vi "senser.vi"(1 "read buffer":string) -> (0 "输出簇":T1)   [LabVIEW 2014]
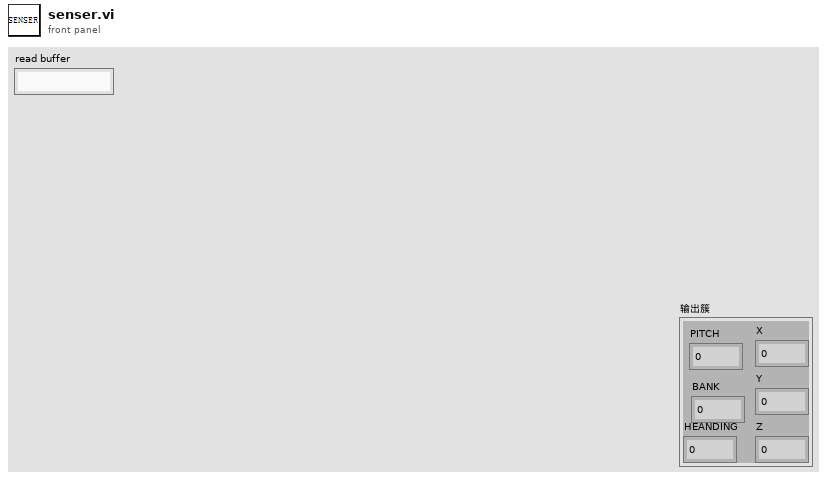
[diagram p1: front panel]
types:
  T1 = cluster{"PITCH":i32, "BANK":i32, "HEANDING":i32, "X":i32, "Y":i32, "Z":i32}
  T2 = cluster{"32位整型":i32, "32位整型":i32, "32位整型":i32, "32位整型":i32, "32位整型":i32, "32位整型":i32}
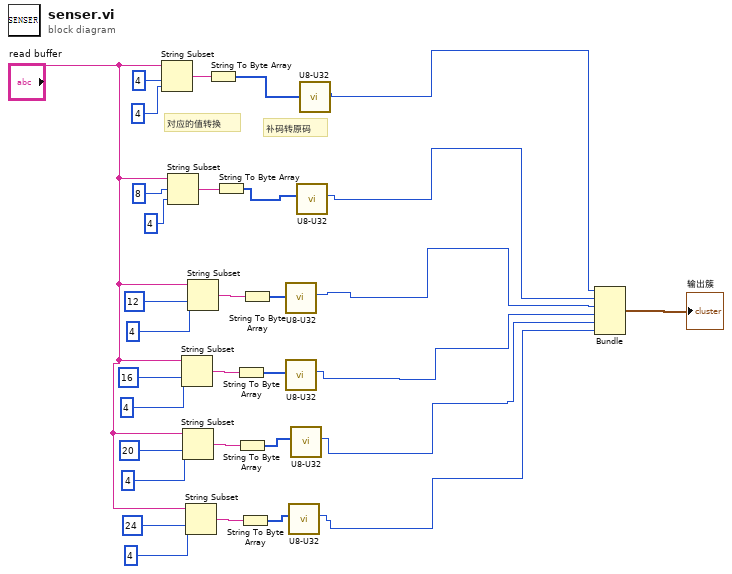
[diagram p0: block diagram]
diagram:
  # "对应的值转换"
  # "补码转原码"
  n1 = String Subset(string="read buffer", offset (0)=4 ("长度（剩余）"), length (rest)=4 ("长度（剩余）")) -> (substring=w16:string)
  n2 = String Subset(string="read buffer", offset (0)=8 ("长度（剩余）"), length (rest)=4 ("长度（剩余）")) -> (substring=w19:string)
  n3 = String Subset(string="read buffer", offset (0)=16 ("长度（剩余）"), length (rest)=4 ("长度（剩余）")) -> (substring=w25:string)
  n4 = String Subset(string="read buffer", offset (0)=20 ("长度（剩余）"), length (rest)=4 ("长度（剩余）")) -> (substring=w28:string)
  n5 = String Subset(string="read buffer", offset (0)=24 ("长度（剩余）"), length (rest)=4 ("长度（剩余）")) -> (substring=w31:string)
  n6 = String Subset(string="read buffer", offset (0)=12 ("长度（剩余）"), length (rest)=4 ("长度（剩余）")) -> (substring=w22:string)
  n7 = String To Byte Array(string=w16) -> (unsigned byte array=w12:u8[])
  n8 = String To Byte Array(string=w19) -> (unsigned byte array=w10:u8[])
  n9 = String To Byte Array(string=w25) -> (unsigned byte array=w2:u8[])
  n10 = String To Byte Array(string=w28) -> (unsigned byte array=w6:u8[])
  n11 = String To Byte Array(string=w31) -> (unsigned byte array=w4:u8[])
  n12 = String To Byte Array(string=w22) -> (unsigned byte array=w8:u8[])
  n13 = call "U8-U32.vi"("数组"=w8) -> ("32位整型"=w7:i32)  [unwired: 8 in, 1 out]
  n14 = call "U8-U32.vi"("数组"=w2) -> ("32位整型"=w1:i32)  [unwired: 8 in, 1 out]
  n15 = call "U8-U32.vi"("数组"=w4) -> ("32位整型"=w3:i32)  [unwired: 8 in, 1 out]
  n16 = call "U8-U32.vi"("数组"=w6) -> ("32位整型"=w5:i32)  [unwired: 8 in, 1 out]
  n17 = call "U8-U32.vi"("数组"=w10) -> ("32位整型"=w9:i32)  [unwired: 8 in, 1 out]
  n18 = call "U8-U32.vi"("数组"=w12) -> ("32位整型"=w11:i32)  [unwired: 8 in, 1 out]
  n19 = Bundle("32位整型"=w11, "32位整型"=w9, "32位整型"=w7, "32位整型"=w1, "32位整型"=w5, "32位整型"=w3) -> (→"输出簇":T2)  [unwired: 1 in]
